vi "Program01.vi"() -> ()   [LabVIEW 2020]
panel:
  out "Waveform Chart":dbl(graph)
  out "Numeric":dbl
  in  "Knob":dbl(knob) scale=0.0..10.0
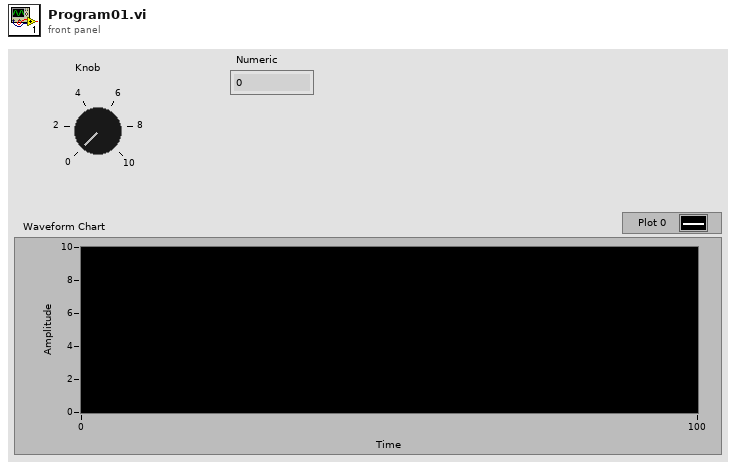
[diagram p1: front panel]
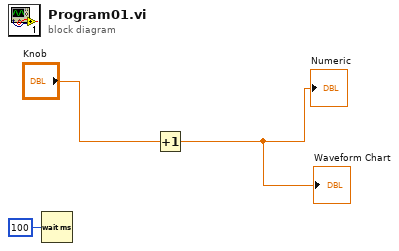
[diagram p0: block diagram]
diagram:
  n1 = Wait (ms)(milliseconds to wait=u32 100) -> ()  [unwired: 1 out]
  n2 = Increment(x="Knob") -> (x+1=→"Numeric" →"Waveform Chart":dbl)
